vi "MacroErrorsFGV.vi"(7 "MacroErrorsFGV_Commands":T2, 8 "Error In":errorcluster, 11 "Error Array IN":T1[](array[typedef])) -> (0 "Error Out":errorcluster, 3 "Error Array OUT":T1[](array[typedef]))   [LabVIEW 2012]
doc: "SciScan 1.2 160622\nThis FGV stores the error descriptions related to macros (read from a file during software init) and can be used to generate errors in a macro code"
uses:
  MacroErrorsFGV_Commands.ctl
  Error Checking/Macro Error Cluster.ctl
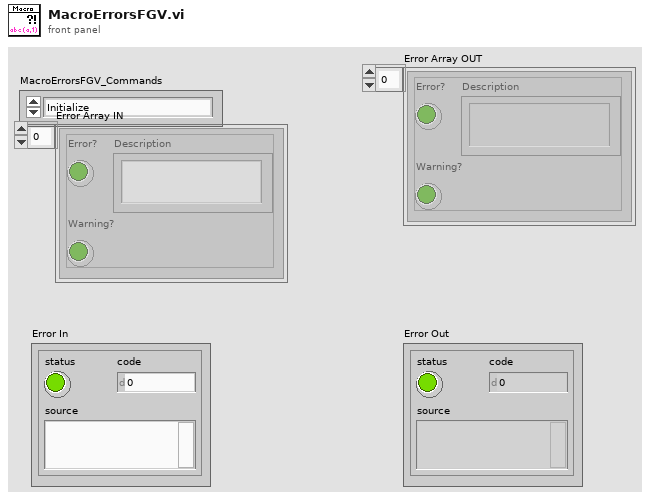
[diagram p1: front panel]
types:
  T1 = typedef "Macro Error Cluster.ctl" = cluster{"Error?":bool, "Description":string, "Warning?":bool}
  T2 = typedef "MacroErrorsFGV_Commands.ctl" = enum16{"Initialize", "Get Error Array", "Set Error Array"}
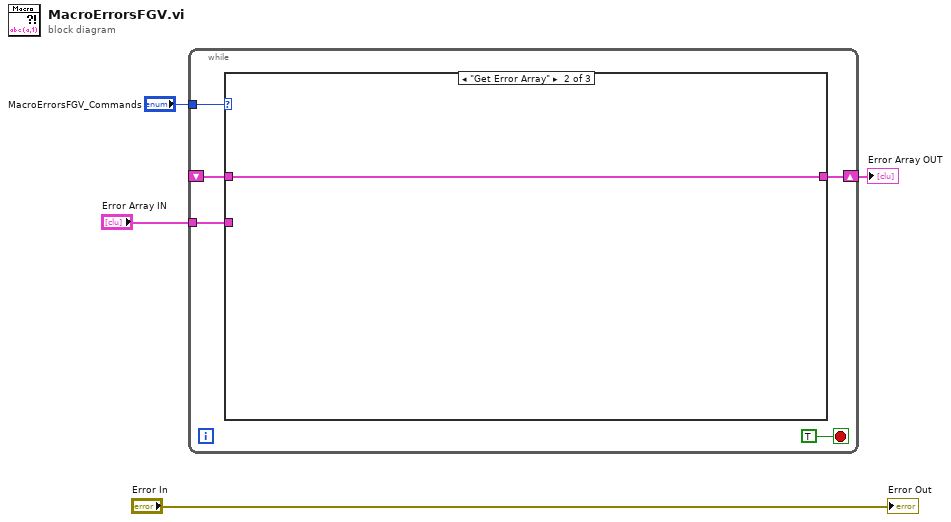
[diagram p0: block diagram]
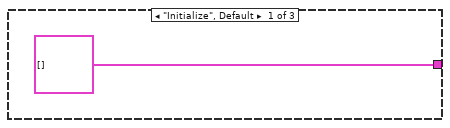
[diagram p2: hidden frame]
diagram:
  n1 = while {
    tunnel: "MacroErrorsFGV_Commands" -> [w9]
    shift-right: [w7] -> w2
    shift-left: _ -> [w6]
    tunnel: "Error Array IN" -> [w5]
    stop <- TRUE stop-if-true
    n2 = case shown="\"Get Error Array\"" w9 {
      tunnel: [T1[] [] w11 w12] -> w7
      tunnel: w6 -> [_ w11 _]
      tunnel: w5 -> [_ _ w12]
      frame "Initialize", Default {
      }
      frame "Get Error Array" {
      }
      frame "Set Error Array" {
      }
    }
  }
  "Error Array OUT" <- w2
  "Error Out" <- "Error In"
